vi "Interpret_Read Device Identification.vi"(8 "error in (no error)":errorcluster, 11 "MB_PDU_resp in":T2={"Function Code"=1, "Data"=[], "RTU_DataBytes"=0}) -> (0 "error out":errorcluster, 1 "DevID Objects":T1[](array[typedef]), 2 "Next Object ID":u8, 3 "Conformity Level":u8)   [LabVIEW 2021, in "MB Master.lvlib"]
doc: "Extracts the data of a PDU request/response pair based on the function code of the response.\n\nReturns an array of device ID objects."
uses:
  <vilib>/Plasmionique/MB Master/MB Master.lvlib
  <vilib>/Plasmionique/MB Master/MB_PDU/MB_PDU_Cluster.ctl
  <vilib>/Plasmionique/MB Master/MB_PDU/MB_DevID Object.ctl
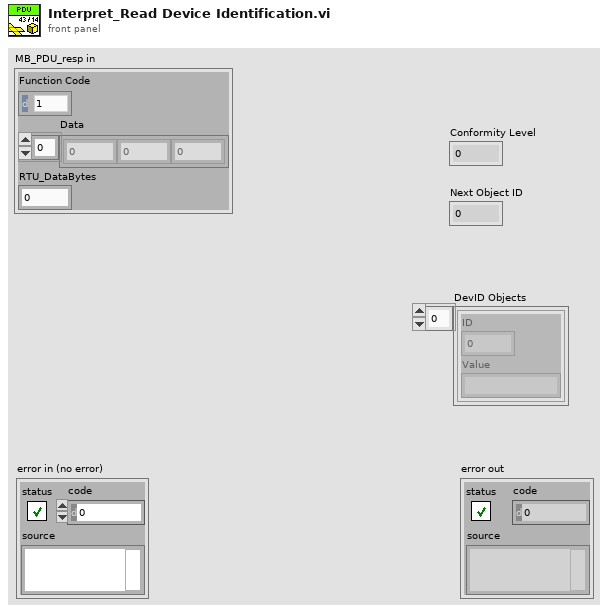
[diagram p1: front panel]
types:
  T1 = typedef "MB Master.lvlib/MB_DevID Object.ctl" = cluster{"ID":u8, "Value":string}
  T2 = typedef "MB Master.lvlib/MB_PDU_Cluster.ctl" = cluster{"Function Code":u8, "Data":u8[], "RTU_DataBytes":i32}
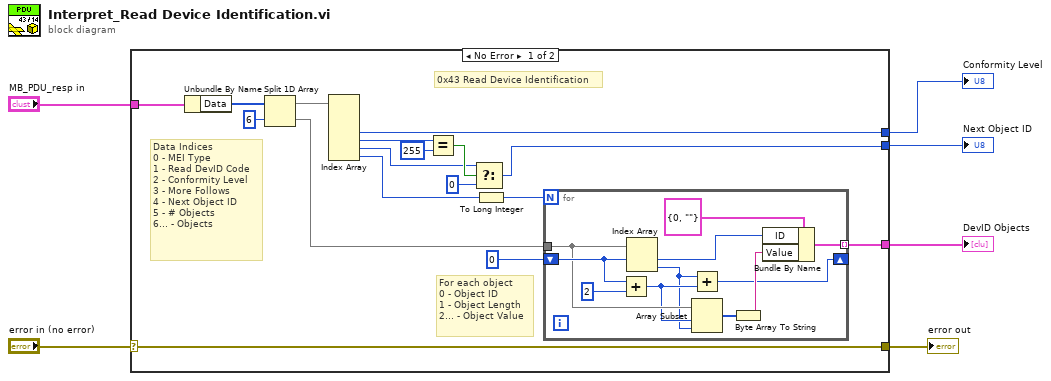
[diagram p0: block diagram]
diagram:
  n1 = case shown="No Error" "error in (no error)" {
    selector: "error in (no error)" -> [w8 w35]
    tunnel: [w8 w35] -> w5
    tunnel: "MB_PDU_resp in" -> [w23 _]
    tunnel: [w22 _] -> w3
    tunnel: [w16 _] -> w2
    tunnel: [w7 _] -> w1
    frame No Error {
      # "For each object\n0 - Object ID\n1 - Object Length\n2... - Object Value"
      # "Data Indices \n0 - MEI Type\n1 - Read DevID Code\n2 - Conformity Level\n3 - More Follows\n4 - Next Object ID\n5 - # Objects\n6... - Objects"
      # "0x43 Read Device Identification"
      n2 = Unbundle By Name(w23) -> ("Data"=w13:u8[])
      n3 = Split 1D Array(array=w13, index=6) -> (first subarray=w11:u8[], second subarray=w10:u8[])
      n4 = Index Array(array=w11) -> (element #3=w22:u8, element #4=w21:u8, element #5=w18:u8, element #6=w15:u8)  [unwired: 6 in, 2 out]
      n5 = Equal?(x=w21, y=u8 255) -> (x = y?=w19:bool)
      n6 = Select(t=w18, s=w19, f=u8 0) -> (s? t:f=w16:u8)
      n7 = To Long Integer(number=w15) -> (32bit integer=w14:i32)
      n8 = for {
        N: w14 -> [_]
        tunnel: w10 -> [w30]
        shift-right: [w25] -> _
        shift-left: 0 -> [w32]
        tunnel: [w24] -> w7 mode=indexing
        n9 = Add(x=w32, y=2) -> (x+y=w27:i32)
        n10 = Index Array(array=w30, index #1=w32) -> (element #1=w33:u8, element #2=w26:u8)  [unwired: 1 in]
        n11 = Add(x=w26, y=w27) -> (x+y=w25:i32)
        n12 = Array Subset(array=w30, index=w27, length=w26) -> (w29:u8[])
        n13 = Byte Array To String(unsigned byte array=w29) -> (string=w28:string)
        n14 = Bundle By Name(cluster=T1 {"ID"=0, "Value"=""} ("DevID Object"), "ID"=w33, "Value"=w28) -> (w24:T1)
      }
    }
    frame Error {
    }
  }
  "error out" <- w5
  "Conformity Level" <- w3
  "Next Object ID" <- w2
  "DevID Objects" <- w1
